vi "Actor Core.vi"(8 "error in":errorcluster, 11 "Log in":refnum<class "Log.lvclass">) -> (0 "error out":errorcluster, 3 "Actor out":refnum<class "Actor.lvclass">)   [LabVIEW 2015, in "AMS UI.lvlib" / "Log.lvclass"]
doc: "(<B>Filename</B>: Actor Framework.lvlib:Actor.lvclass:Actor Core.vi)\n\nReceives messages to the actor, reacts to them, and initiates any error handling that may shut the actor down.\n\nDescendant classes may override this VI to append parallel tasks for the actor to complete while it handles messages. Overrides use the Call Parent Method node."
uses:
  Log.lvclass
  <vilib>/ActorFramework/Actor/Actor.lvclass
  Log.lvclass/Log.ctl
  <vilib>/ActorFramework/Actor/Actor.lvclass/Actor.ctl
  <vilib>/ActorFramework/Message Enqueuer/Message Enqueuer.lvclass/Message Enqueuer.ctl
  Log Messages/Log Message Msg/Log Message Msg.lvclass/Log Message Msg.ctl
  <vilib>/ActorFramework/Message Enqueuer/Init from Existing Queue.vi
  <vilib>/ActorFramework/Message Enqueuer/Enqueue.vi
  <vilib>/ActorFramework/Message Priority Queue/Priority Enqueue.vi
  <vilib>/ActorFramework/Message Enqueuer/Message Enqueuer.lvclass
  Log Messages/Log Message Msg/Log Message Msg.lvclass
  Log Messages/Log to Clipboard Msg/Log to Clipboard Msg.lvclass
  AMS Gas Actor/AMS Gas Actor.lvclass
  eActor/eActor.lvclass
panel:
  in  "Copy Button":bool
  in  "Clear Button":bool
  out "Listbox":i32(listbox)
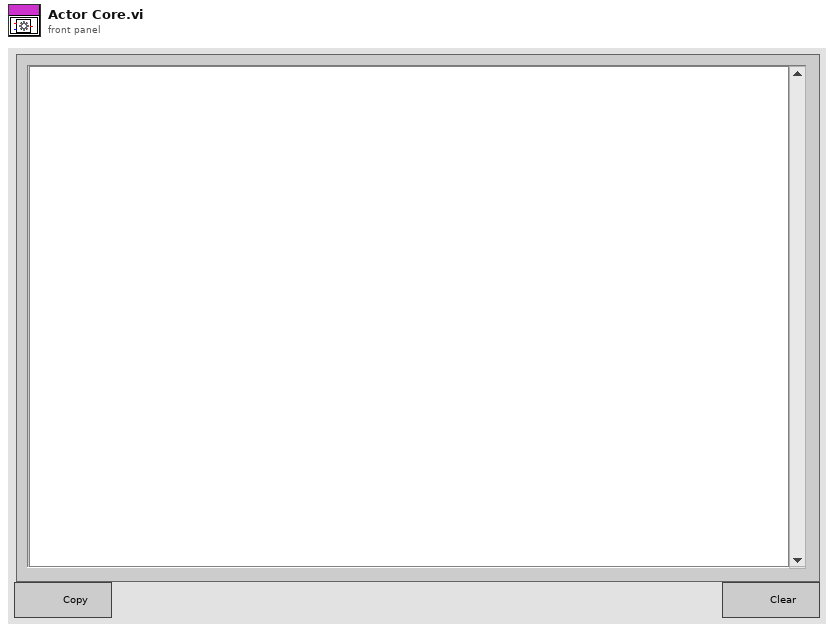
[diagram p1: front panel]
types:
  T1 = enum32{"Invalid", "Standard", "Closed", "Hidden", "Minimized", "Maximized"}
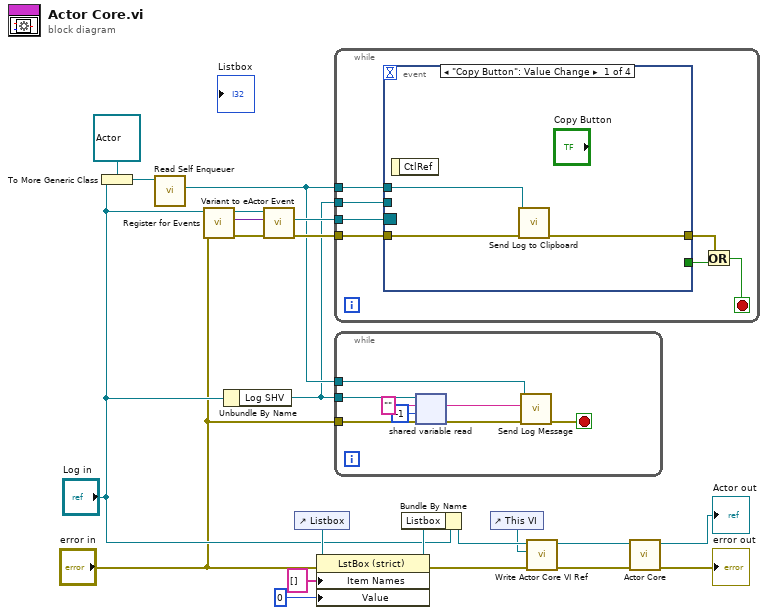
[diagram p0: block diagram]
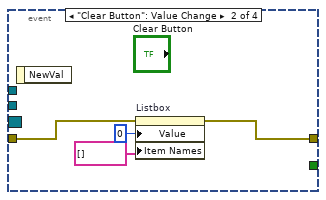
[diagram p2: hidden frame]
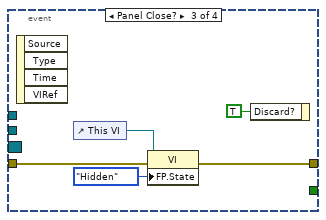
[diagram p3: hidden frame]
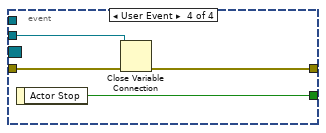
[diagram p4: hidden frame]
diagram:
  n1 = To More Generic Class(target class=refnum<class "Actor.lvclass"> refnum ("Actor"), reference="Log in") -> (generic class reference=w20:refnum<class "Actor.lvclass">)
  n2 = call <vilib>:"Read Self Enqueuer.vi"("Actor"=w20) -> ("Self Enqueuer"=w3:refnum<class "Message Enqueuer.lvclass">)  [unwired: 10 in]
  n3 = call-dynamic "Register for Events.vi"("error in (no error)"="error in", "eActor in"="Log in") -> ("error out"=w13:errorcluster, "Event Registration Refnum"=w12:variant, "eActor out"=w11:refnum<class "Log.lvclass">)  [unwired: 7 in]
  n4 = Unbundle By Name("Log in") -> ("Log SHV"=w2:refnum<k21>)
  n5 = call "Variant to eActor Event.vi"("error in (no error)"=w13, "Variant"=w12, "eActor in"=w11) -> ("error out"=w9:errorcluster, "Event Registration Refnum"=w10:refnum<event-registration>)  [unwired: 6 in, 1 out]
  n6 = control-ref of="Listbox"() -> (w15:refnum<vi>)
  n7 = property class="LstBox (strict)"(reference=w15, error in="error in", "Item Names"=string[] [], "Value"=0) -> (reference out=w14:refnum<vi>, error out=w7:errorcluster)
  n8 = while {
    tunnel: w9 -> [w28]
    tunnel: w10 -> [w29]
    tunnel: w3 -> [w26]
    tunnel: w2 -> [w23]
    stop <- w24 stop-if-true
    n9 = event shown="[0] \"Copy Button\": Value Change" {
      selector: w29 -> [_ _ _ _]
      dyn-events: _ -> [_ _ _ _]
      timeout: _ -> [_ _ _ _]
      tunnel: w28 -> [w32 w33 w40 w44]
      tunnel: [_ _ _ w45] -> w27
      tunnel: w26 -> [w31 _ _ _]
      tunnel: [w30 w36 w37 w43] -> w25
      tunnel: w23 -> [_ _ _ w42]
      event "Copy Button": Value Change {
        n10 = event-data() -> ()  [unwired: 1 in, 1 out]
        n11 = call "Send Log to Clipboard.vi"("error in (no error)"=w32, "Message Enqueuer"=w31) -> ("error out"=w30:errorcluster)  [unwired: 8 in, 1 out]
      }
      event "Clear Button": Value Change {
        n12 = event-data() -> ()  [unwired: 1 in, 1 out]
        n13 = property on="Listbox" class="LstBox (strict)"(error in=w33, "Value"=0 ("Listbox"), "Item Names"=string[] []) -> (error out=w36:errorcluster)  [unwired: 1 in, 1 out]
      }
      event Panel Close? {
        n14 = event-data() -> ()  [unwired: 1 in, 4 out]
        n15 = control-ref of="This VI"() -> (w39:refnum<vi>)
        n16 = property class="VI"(reference=w39, error in=w40, "FP.State"=T1."Hidden" ("Front Panel Window:State")) -> (error out=w37:errorcluster)  [unwired: 1 out]
        n17 = event-data("Discard?"=TRUE) -> ()  [unwired: 1 in, 1 out]
      }
      event User Event {
        n18 = event-data() -> ("Actor Stop"=w45:bool)  [unwired: 1 in]
        n19 = Close Variable Connection(8:w44, 11:w42) -> (0:w43:errorcluster)
      }
    }
    n20 = Or(x=w25, y=w27) -> (x .or. y?=w24:bool)
  }
  n21 = while {
    tunnel: w2 -> [w51]
    tunnel: "error in" -> [w50]
    tunnel: w3 -> [w53]
    stop <- w52 stop-if-true
    n22 = shared-variable-read(w51, w50, "", -1 ("timeout ms")) -> (w49:errorcluster, w46:string)  [unwired: 3 out]
    n23 = call "Send Log Message.vi"("error in (no error)"=w49, "String"=w46, "Message Enqueuer"=w53) -> ("error out"=w52:errorcluster)  [unwired: 7 in, 1 out]
  }
  n24 = Bundle By Name(cluster="Log in", "Listbox"=w14) -> (w18:refnum<class "Log.lvclass">)
  n25 = control-ref of="This VI"() -> (w1:refnum<vi>)
  n26 = call "Write Actor Core VI Ref.vi"("error in (no error)"=w7, "Actor Core VI Ref"=w1, "AMS Gas Actor in"=w18) -> ("error out"=w6:errorcluster, "AMS Gas Actor out"=w8:refnum<class "Log.lvclass">)  [unwired: 7 in]
  n27 = call-parent "Actor Core.vi"("error in"=w6, "Actor in"=w8) -> ("error out"=→"error out":errorcluster, "Actor out"=→"Actor out":refnum<class "Actor.lvclass">)  [unwired: 8 in]
